vi "写串口.vi"(9 "delay before read (ms)":u32=100 caption="读取前延时(ms)", 11 "写入缓冲区":string) -> (1 "bytes read":u32 caption="读取的字节", 3 "read string":string caption="读取字符串")   [LabVIEW 2012]
uses:
  <vilib>/Instr/_visa.llb/VISA Configure Serial Port (Instr).vi
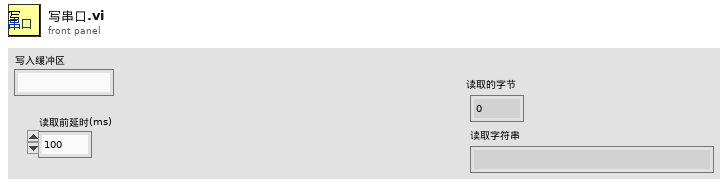
[diagram p1: front panel]
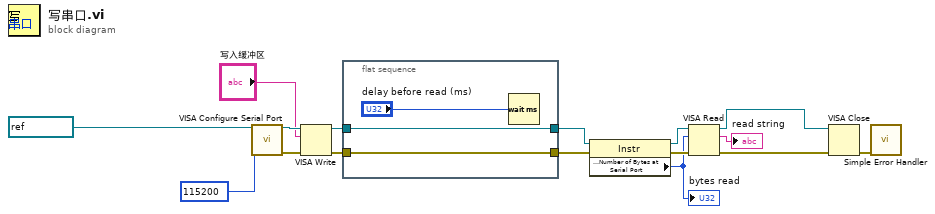
[diagram p0: block diagram]
diagram:
  n1 = call-poly "VISA Configure Serial Port"("VISA resource name"=refnum<visa-resource-name> "COM1", "baud rate (9600)"=u32 115200) -> ("VISA resource name out"=w15:refnum<visa-resource-name>, "error out"=w13:errorcluster)  [unwired: 12 in]
  n2 = VISA Write(VISA resource name=w15, write buffer="写入缓冲区", error in (no error)=w13) -> (VISA resource name out=w6:refnum<visa-resource-name>, error out=w9:errorcluster)  [unwired: 1 out]
  n3 = flat-sequence {
    tunnel: w9 -> [w18]
    tunnel: [w18] -> w8
    tunnel: [w17] -> w7
    tunnel: w6 -> [w17]
    frame #0 {
      n4 = Wait (ms)(milliseconds to wait="delay before read (ms)") -> ()  [unwired: 1 out]
    }
  }
  n5 = property class="Instr"(reference=w7, error in=w8) -> (reference out=w5:refnum<visa-resource-name>, error out=w4:errorcluster, "Serial Settings:Number of Bytes at Serial Port"=w2:u32)
  "bytes read" <- w2
  n6 = VISA Read(VISA resource name=w5, byte count=w2, error in (no error)=w4) -> (VISA resource name out=w11:refnum<visa-resource-name>, read buffer=→"read string":string, error out=w12:errorcluster)  [unwired: 1 out]
  n7 = VISA Close(VISA resource name=w11, error in (no error)=w12) -> (error out=w10:errorcluster)
  n8 = call <vilib>:"Simple Error Handler.vi"("error in (no error)"=w10) -> ()  [unwired: 1 in, 8 out]
